vi "SetExposureTimeSD.vi"(2 "error in (no error)":errorcluster, 3 "time":sgl format="%.2f") -> (0 "error out":errorcluster, 1 "DLL error code":u32)   [LabVIEW 2015]
doc: "This function will set the exposure time to the nearest valid value not less than the given value. The actual exposure time used is obtained by <B>GetAcquisitionTimings</B>. See section on Acquisition Modes for further details.\n\n<B>Parameter:</B>\ntime - the exposure time in seconds.\n\n<B>Error codes:</B>\nDRV_SUCCESS - Exposure time accepted.\nDRV_NOT_INITIALIZED - System not initialized.\nDRV_ACQUIRING - Acquisition in progress.\nDRV_P1INVALID - Exposure Time invalid.\n\n<B>NOTES:</B>\n<B>If the current acquisition mode is Single-track, Multi-Track or Image then this function will actually set the shutter time. The actual exposure time used is obtained from GetAcquisitionTimings.</B>"
uses:
  DLL/atmcd32d.dll
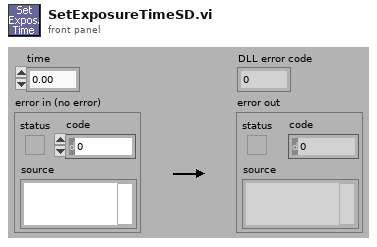
[diagram p1: front panel]
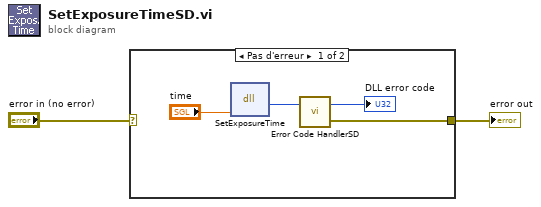
[diagram p0: block diagram]
diagram:
  n1 = case shown="Pas d'erreur" "error in (no error)" {
    selector: "error in (no error)" -> [_ w7]
    tunnel: [w5 w7] -> w1
    frame No Error {
      n2 = dll-call lib="G:/SD/TRANCON-2015/DLL/Atmcd32d.dll" fn="SetExposureTime"("time"="time") -> ("return type"=w6:u32)  [unwired: 4 in, 2 out]
      n3 = call "Error Code HandlerSD.vi"("DLL error code"=w6) -> ("error out"=w5:errorcluster, "dup DLL error code"=→"DLL error code":u32)  [unwired: 1 in]
    }
    frame Error {
    }
  }
  "error out" <- w1
